vi "timming_array_to_digital_waveform.vi"(3 "delay array":dbl[](array[numeric]) format="%#_6e", 4 "resolution":i32=100) -> (0 "digital waveform":digitalwaveform(waveform)={"t0"=timestamp(0 s since 1904-01-01), "dt"=0.0, "Y"={"transitions"=[], "data"=[]}, "error"={"status"=FALSE, "code"=37421928, "source"=""}})   [LabVIEW 2011]
doc: "takes the timing info recieved from the DG645 Delay generator and transforms it into a digital waveform graph.\nMakes sure, all timings are setup in reference to t0!"
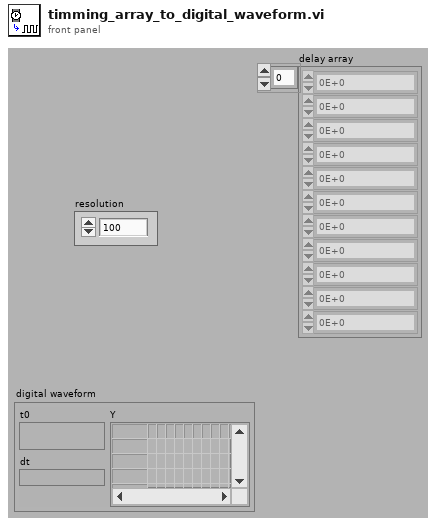
[diagram p1: front panel]
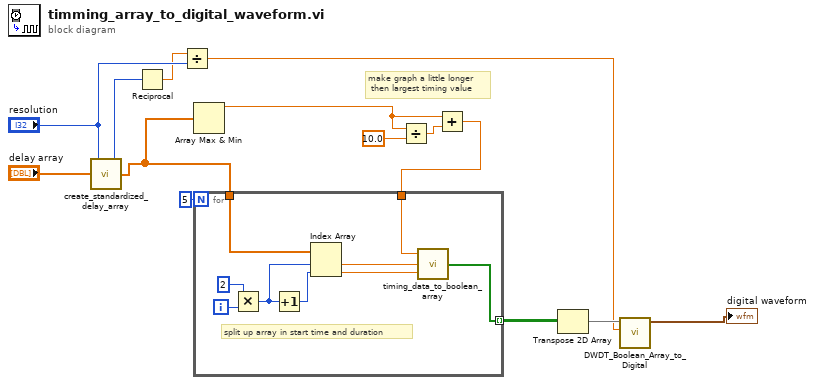
[diagram p0: block diagram]
diagram:
  # "make graph a little longer\n then largest timing value"
  n1 = call "create_standardized_delay_array.vi"("delay array"="delay array", "resolution"="resolution") -> ("standardize array"=w7:dbl[], "multiplier"=w4:i32)  [unwired: 2 in]
  n2 = Reciprocal(x=w4) -> (1/x=w3:dbl)
  n3 = Divide(x=w3, y="resolution") -> (x/y=w5:dbl)
  n4 = Array Max & Min(array=w7) -> (max value=w9:dbl)  [unwired: 3 out]
  n5 = Divide(x=w9, y=10.0) -> (x/y=w1:dbl)
  n6 = Add(x=w9, y=w1) -> (x+y=w10:dbl)
  n7 = for {
    N: 5 -> [_]
    tunnel: [w21] -> w13 mode=indexing
    tunnel: w10 -> [w20]
    tunnel: w7 -> [w15]
    i -> [w23]
    # "split up array in start time and duration"
    n8 = Multiply(x=2, y=w23) -> (x*y=w16:i32)
    n9 = Increment(x=w16) -> (x+1=w19:i32)
    n10 = Index Array(array=w15, index #1=w16, index #2=w19) -> (element #1=w18:dbl, element #2=w17:dbl)
    n11 = call "timing_data_to_boolean_array.vi"("end time [s]"=w17, "start time [s]"=w18, "overall length [s]"=w20) -> ("boolean timing array"=w21:bool[])  [unwired: 1 in]
  }
  n12 = Transpose 2D Array(2D array=w13) -> (transposed array=w12:bool[][])
  n13 = call "DWDT_Boolean_Array_to_Digital.vi"("delta t"=w5, "boolean array"=w12) -> ("digital waveform"=→"digital waveform":digitalwaveform)  [unwired: 8 in, 1 out]
